vi "ESA_Data_Analysis_Global_VIs.vi"() -> ()   [LabVIEW 2015]
panel:
  in  "Add Chs":bool
  in  "offset":dbl format="%#_13g"
  out "Cursors":T1
  out "Total Int.":dbl caption="Total Integration Duration (s)" format="%#.3p"
  out "Tail Int.":dbl caption="Tail Integration Duration (s)" format="%#.3p"
  in  "Discr. Limit":dbl=2.5
  in  "Graph resolution":dbl=5.0
  in  "Listbox":i32[](listbox) caption="ListBox"
  out "tdms file out":refnum<k34>
  out "group names":string[](array[string])
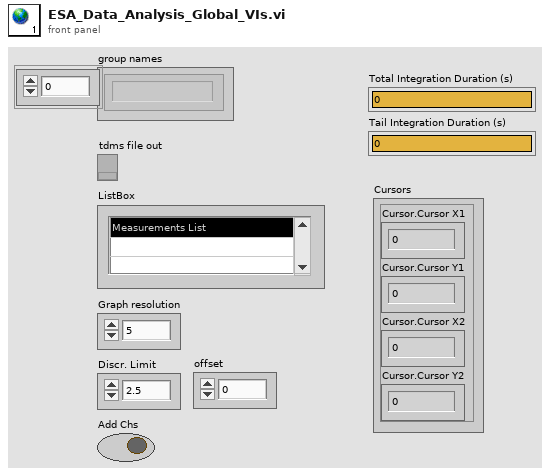
[diagram p1: front panel]
types:
  T1 = cluster{"Cursor.Cursor X1":dbl, "Cursor.Cursor Y1":dbl, "Cursor.Cursor X2":dbl, "Cursor.Cursor Y2":dbl}
diagram:
